vi "ES Randomize Measurements.vi"(10 "DeviceID":T2) -> (3 "ES_Measurement Array out":T1[](array[typedef]))   [LabVIEW 2018, in "IED Test Framework.lvlib" / "IED Test.lvclass"]
uses:
  IED Test.lvclass
  <vilib>/ORNL/CSEISMIC DDS/CSEISMIC DDS Base/Data Types/Controls/DeviceID.ctl
  <vilib>/ORNL/CSEISMIC DDS/CSEISMIC DDS Base/Data Types/ES_Measurement.ctl
  <vilib>/ORNL/CSEISMIC DDS/CSEISMIC DDS Base/CSEISMIC DDS.lvclass
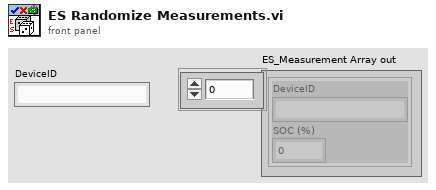
[diagram p1: front panel]
types:
  T1 = typedef "CSEISMIC DDS.lvlib/CSEISMIC DDS.lvclass/ES_Measurement.ctl" = cluster{"DeviceID":T2, "SOC (%)":dbl}
  T2 = typedef "CSEISMIC DDS.lvlib/CSEISMIC DDS.lvclass/DeviceID.ctl" = string
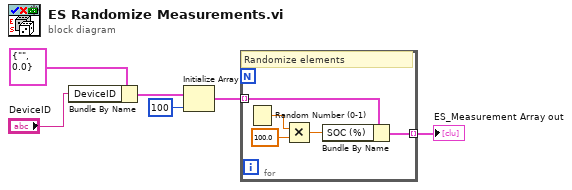
[diagram p0: block diagram]
diagram:
  n1 = Bundle By Name(cluster=T1 {"DeviceID"="", "SOC (%)"=0.0} ("ES_Measurement"), "DeviceID"="DeviceID") -> (w5:T1)
  n2 = Initialize Array(w5, 100 ("dimension size")) -> (w2:T1[])
  n3 = for {
    tunnel: w2 -> [w11] mode=indexing
    tunnel: [w10] -> w1 mode=indexing
    # "Randomize elements"
    n4 = Random Number (0-1)() -> (number: 0 to 1=w9:dbl)
    n5 = Multiply(x=w9, y=100.0) -> (x*y=w7:dbl)
    n6 = Bundle By Name(cluster=w11, "SOC (%)"=w7) -> (w10:T1)
  }
  "ES_Measurement Array out" <- w1
